vi "svfa_Peak Rough Search Indices.vi"(0 "x":dbl[](array[numeric]) format="%.5e", 1 "threshold":dbl=-inf format="%.2f") -> (5 "peak indices":i32[](array[numeric]))   [LabVIEW 2017]
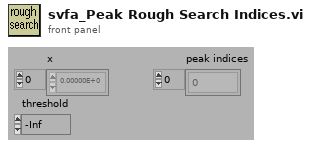
[diagram p1: front panel]
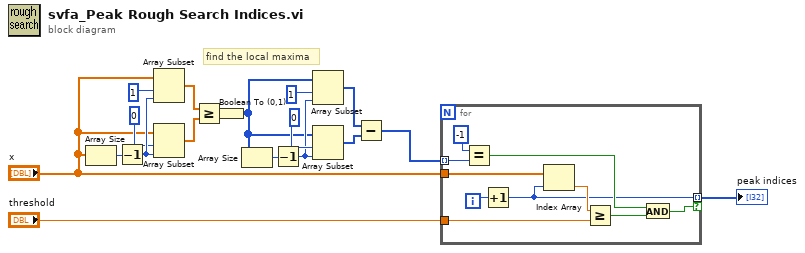
[diagram p0: block diagram]
diagram:
  # "find the local maxima"
  n1 = Array Size(array="x") -> (size(s)=w17:i32)
  n2 = Decrement(x=w17) -> (x-1=w16:i32)
  n3 = Array Subset(array="x", index=1, length=w16) -> (w13:dbl[])
  n4 = Array Subset(array="x", index=0, length=w16) -> (w12:dbl[])
  n5 = Greater Or Equal?(x=w13, y=w12) -> (x >= y?=w11:bool[])
  n6 = Boolean To (0,1)(Boolean=w11) -> (0, 1=w6:i16[])
  n7 = Array Size(array=w6) -> (size(s)=w7:i32)
  n8 = Decrement(x=w7) -> (x-1=w8:i32)
  n9 = Array Subset(array=w6, index=1, length=w8) -> (w5:i16[])
  n10 = Array Subset(array=w6, index=0, length=w8) -> (w4:i16[])
  n11 = Subtract(x=w5, y=w4) -> (x-y=w3:i16[])
  n12 = for {
    tunnel: w3 -> [w25] mode=indexing
    tunnel: "x" -> [w27]
    tunnel: "threshold" -> [w26]
    tunnel: [w20] -> w1 mode=indexing if=w19
    i -> [w24]
    n13 = Equal?(x=i16 -1, y=w25) -> (x = y?=w21:bool)
    n14 = Increment(x=w24) -> (x+1=w20:i32)
    n15 = Index Array(array=w27, index=w20) -> (element=w23:dbl)
    n16 = Greater Or Equal?(x=w23, y=w26) -> (x >= y?=w22:bool)
    n17 = And(x=w21, y=w22) -> (x .and. y?=w19:bool)
  }
  "peak indices" <- w1
